vi "mpcController.vi"(8 "error in (no error)":errorcluster, 10 "RobotRef in":refnum<class "Robot.lvclass">[](array[class]), 11 "Game in":refnum<class "Game.lvclass">) -> (0 "error out":errorcluster, 2 "RobotRef out":refnum<class "Robot.lvclass">[](array[class]), 3 "Game out":refnum<class "Game.lvclass">)   [LabVIEW 2021, in "Game.lvclass"]
uses:
  Game.lvclass
  Robot_class/Robot.lvclass
  C:/Users/anton/Desktop/RoboIME/IC/SSL_AI/Object_class/Object.lvclass
  Object_class/Object.lvclass/Object.ctl
  Robot_class/Robot.lvclass/Robot.ctl
  <vilib>/Analysis/coordinate.llb/2D Cartesian Coordinate Rotation (Scalar).vi
  Object_class/Read x.vi
  Object_class/Read y.vi
  Robot_class/Read orientation.vi
  Robot_class/Read dest_x.vi
  Robot_class/Read dest_y.vi
  Robot_class/Read dest_orientation.vi
  Robot_class/Write v_tang.vi
  Robot_class/Write v_norm.vi
  Robot_class/Write v_ang.vi
  <vilib>/Analysis/NI_AALPro.lvlib
panel:
  in  "y":i32
  out "Waveform Chart":dbl[](graph)
  out "error out 2":errorcluster
  out "return value 3":dbl[](array[numeric])
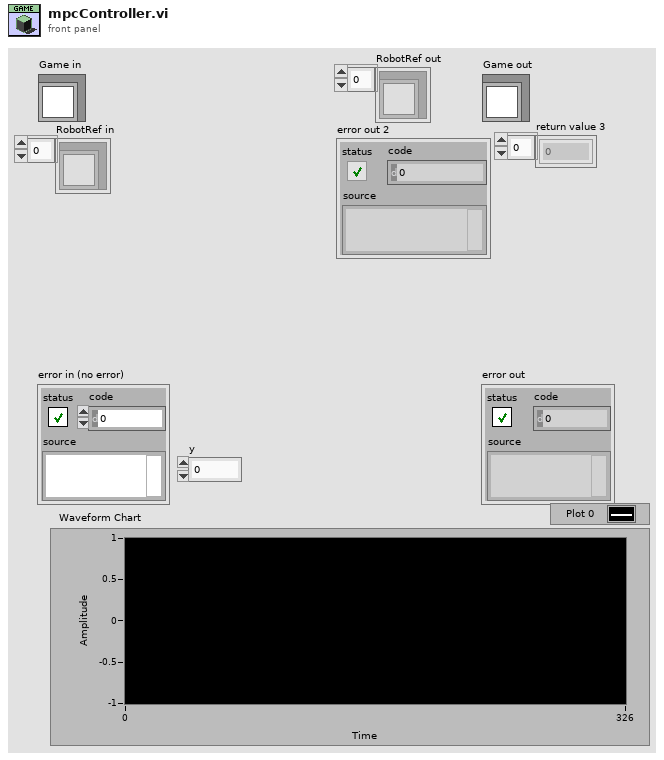
[diagram p1: front panel]
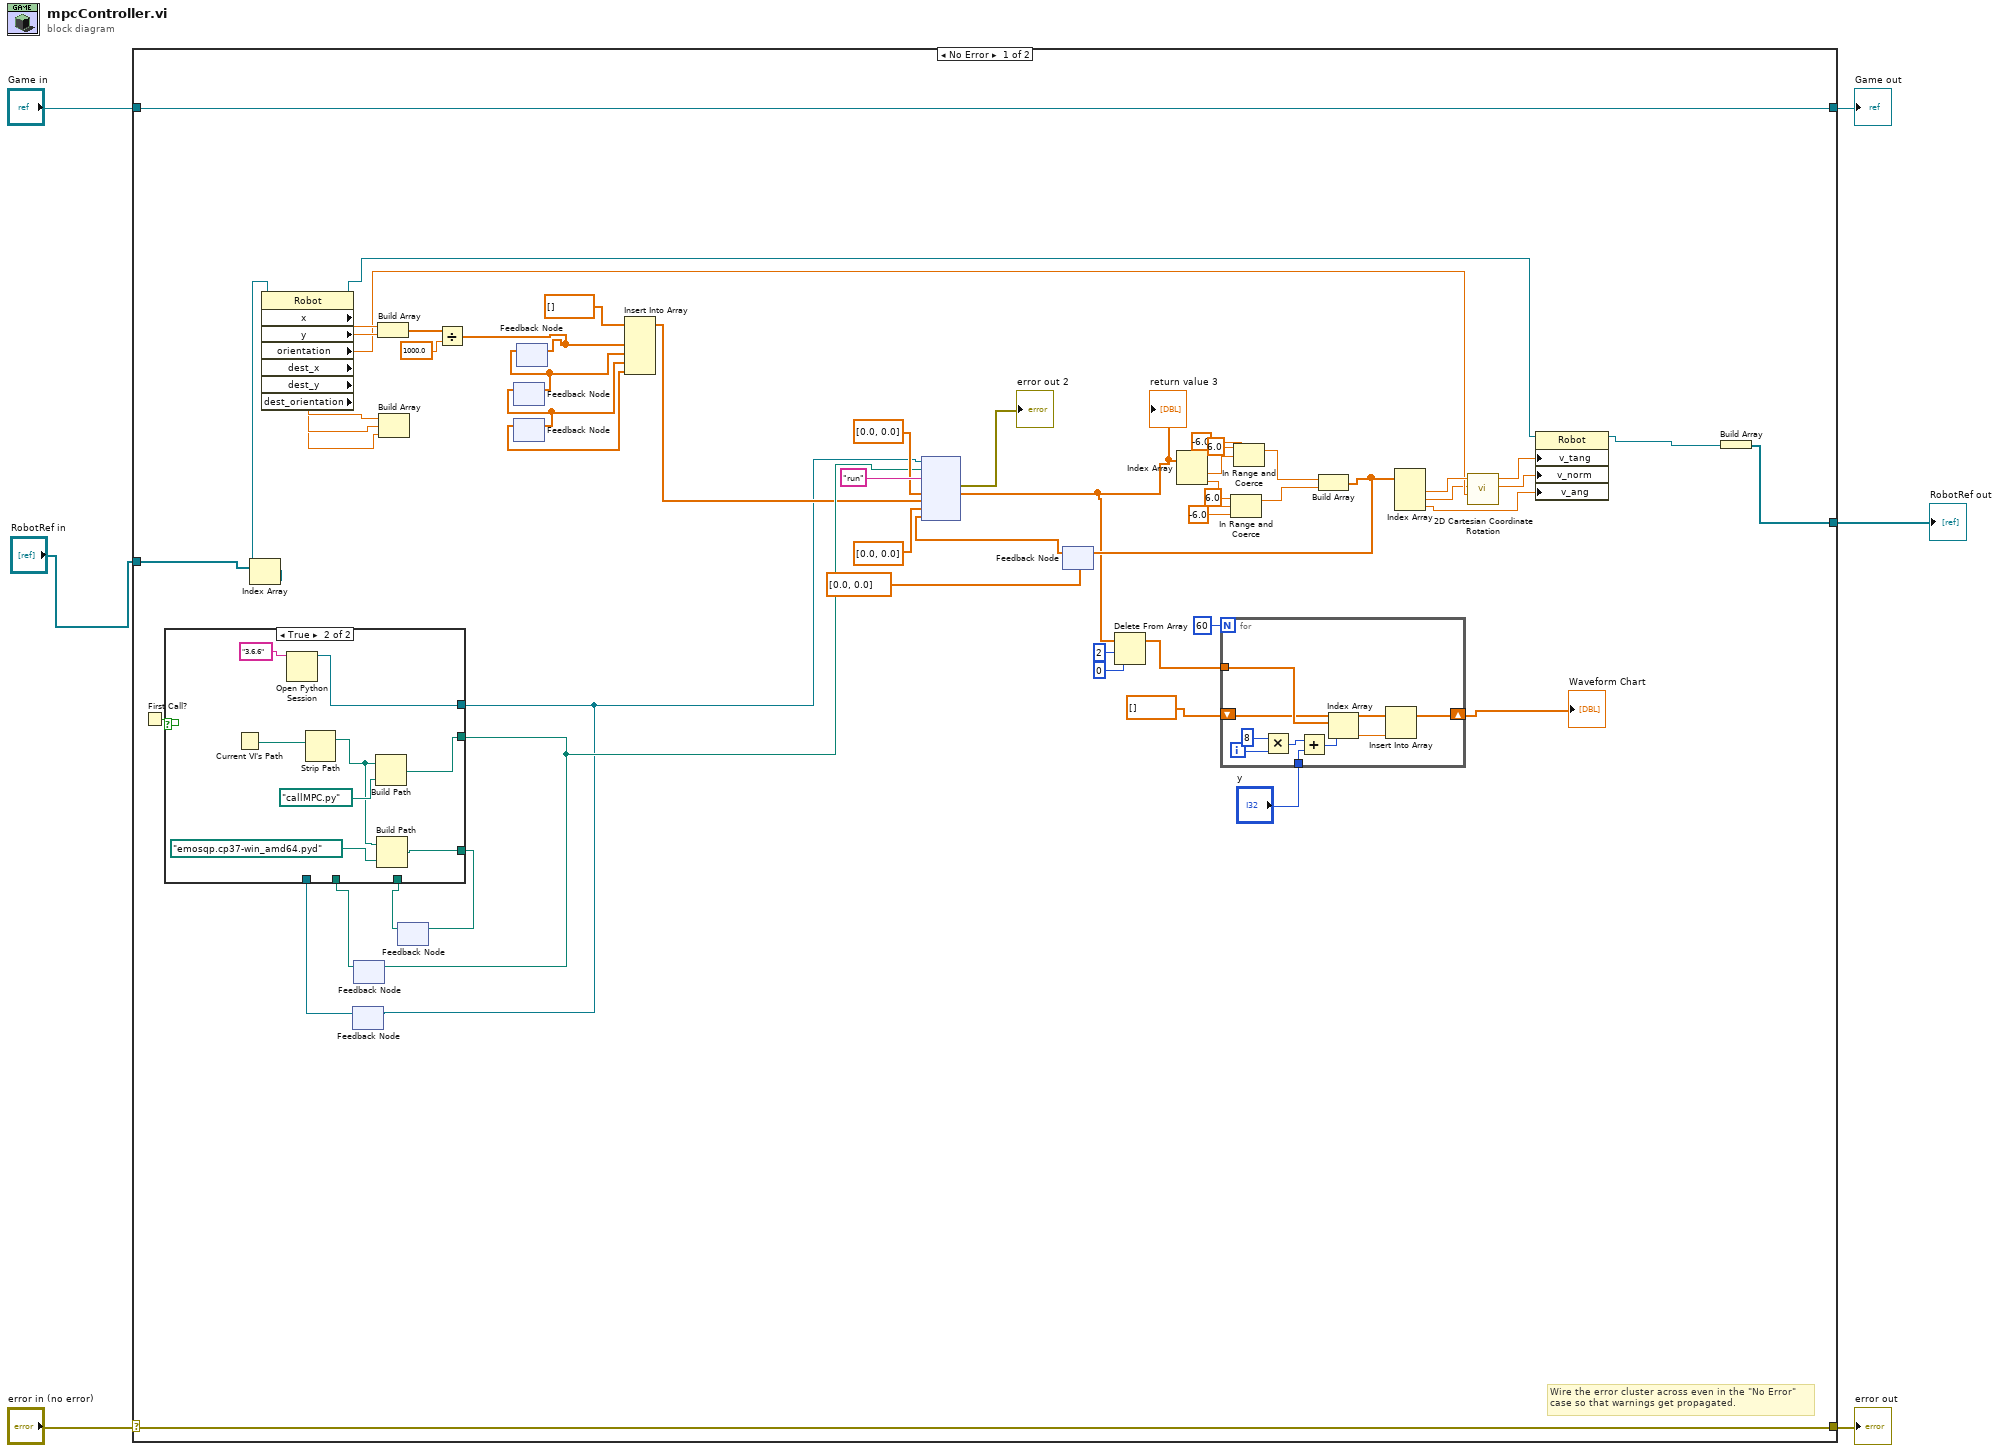
[diagram p0: block diagram]
diagram:
  n1 = case shown="No Error" "error in (no error)" {
    selector: "error in (no error)" -> [w61 w84]
    tunnel: [w61 w84] -> w5
    tunnel: [w62 w83] -> w3
    tunnel: "Game in" -> [w62 w83]
    tunnel: "RobotRef in" -> [w60 _]
    tunnel: [w58 _] -> w2
    frame No Error {
      # "Wire the error cluster across even in the \"No Error\"\ncase so that warnings get propagated."
      n2 = First Call?() -> (First Call?: T/F=w41:bool)
      n3 = Index Array(array=w60) -> (element=w43:refnum<class "Robot.lvclass">)  [unwired: 1 in]
      n4 = property class="Robot"(reference=w43) -> (reference out=w46:refnum<class "Robot.lvclass">, "x"=w57:dbl, "y"=w56:dbl, "orientation"=w50:dbl, "dest_x"=w55:dbl, "dest_y"=w54:dbl, "dest_orientation"=w53:dbl)  [unwired: 1 in, 1 out]
      n5 = feedback #1() -> (w39:refnum<k35>)  [unwired: 1 in]
      n6 = feedback #2() -> (w40:path)  [unwired: 1 in]
      n7 = Build Array(w57, w56) -> (w12:dbl[])
      n8 = Build Array(w55, w54, w53) -> ()  [unwired: 1 out]
      n9 = feedback #3() -> (w9:path)  [unwired: 1 in]
      n10 = case shown="True" w41 {
        tunnel: [w74 w82] -> w38
        tunnel: [w73 w78] -> w7
        tunnel: w40 -> [w74 _]
        tunnel: w39 -> [w73 _]
        tunnel: [w72 w75] -> w8
        tunnel: w9 -> [w72 _]
        frame False {
        }
        frame True {
          n11 = Current VI's Path() -> (path=w80:path)
          n12 = Open Python Session(python version="3.6.6" ("Python version")) -> (session out=w78:refnum<k35>)  [unwired: 2 in, 1 out]
          n13 = Strip Path(path=w80) -> (stripped path=w76:path)  [unwired: 1 out]
          n14 = Build Path(base path=w76, name or relative path=path "callMPC.py" ("module path")) -> (appended path=w82:path)
          n15 = Build Path(base path=w76, name or relative path=path "emosqp.cp37-win_amd64.pyd" ("module path")) -> (appended path=w75:path)
        }
      }
      n16 = feedback-in #1(w7) -> ()
      n17 = feedback-in #2(w38) -> ()
      n18 = feedback-in #3(w8) -> ()
      n19 = Divide(x=w12, y=1000.0) -> (x/y=w10:dbl[])
      n20 = feedback #4() -> (w17:dbl[])  [unwired: 1 in]
      n21 = feedback #5() -> (w35:dbl[])  [unwired: 1 in]
      n22 = feedback-in #5(w17) -> ()
      n23 = feedback-in #6(w10) -> ()
      n24 = feedback #6() -> (w18:dbl[])  [unwired: 1 in]
      n25 = feedback-in #4(w18) -> ()
      n26 = Insert Into Array(array=dbl[] [], new element #1=w10, new element #2=w18, new element #3=w17, new element #4=w35) -> (w34:dbl[])  [unwired: 1 in]
      n27 = feedback #7(dbl[] [0.0, 0.0]) -> (w15:dbl[])
      n28 = node(w7, w38, "run" ("function name"), dbl[] [0.0, 0.0], w34, dbl[] [0.0, 0.0] ("appended array"), w15) -> (→"error out 2":errorcluster, w25:dbl[])  [unwired: 4 in, 3 out]
      "return value 3" <- w25
      n29 = Delete From Array(array=w25, length=2, index=0) -> (array with subset deleted=w21:dbl[])  [unwired: 1 out]
      n30 = Index Array(array=w25) -> (element #1=w33:dbl, element #2=w32:dbl)  [unwired: 2 in]
      n31 = for {
        N: 60 -> [_]
        tunnel: w21 -> [w69]
        shift-right: [w66] -> w13
        shift-left: dbl[] [] ("array") -> [w67]
        tunnel: "y" -> [w63]
        i -> [w71]
        n32 = Multiply(x=8, y=w71) -> (x*y=w65:i32)
        n33 = Add(x=w65, y=w63) -> (x+y=w64:i32)
        n34 = Index Array(array=w69, index=w64) -> (element=w68:dbl)
        n35 = Insert Into Array(array=w67, new element=w68) -> (w66:dbl[])  [unwired: 1 in]
      }
      "Waveform Chart" <- w13
      n36 = In Range and Coerce(upper limit=6.0, x=w32, lower limit=-6.0) -> (coerced(x)=w27:dbl)  [unwired: 1 out]
      n37 = In Range and Coerce(upper limit=6.0, x=w33, lower limit=-6.0) -> (coerced(x)=w26:dbl)  [unwired: 1 out]
      n38 = Build Array(w26, w27) -> (w45:dbl[])
      n39 = feedback-in #7(w45) -> ()
      n40 = Index Array(array=w45) -> (element #1=w51:dbl, element #2=w14:dbl, element #3=w47:dbl)  [unwired: 3 in]
      n41 = call-poly <vilib>:"2D Cartesian Coordinate Rotation.vi"("theta"=w50, "y"=w14, "x"=w51) -> ("y out"=w48:dbl, "x out"=w49:dbl)  [unwired: 6 in, 1 out]
      n42 = property class="Robot"(reference=w46, "v_tang"=w49, "v_norm"=w48, "v_ang"=w47) -> (reference out=w59:refnum<class "Robot.lvclass">)  [unwired: 1 in, 1 out]
      n43 = Build Array(w59) -> (w58:refnum<class "Robot.lvclass">[])
    }
    frame Error {
    }
  }
  "error out" <- w5
  "Game out" <- w3
  "RobotRef out" <- w2
